vi "XYgraphBuffer.vi"(8 "Size":i32=100, 11 "X-Y Coord":dbl[](array[numeric])=[0.0, 0.0]) -> (3 "ToXYGraph":T1(array[cluster]))   [LabVIEW 2010, in "kevLib2011.lvlib"]
uses:
  kevLib2011.lvlib
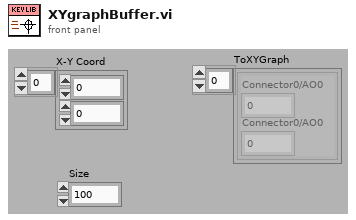
[diagram p1: front panel]
types:
  T1 = cluster{"Connector0/AO0":dbl, "Connector0/AO0":dbl}[]
  T2 = cluster{"Connector0/AO0":dbl, "Connector0/AO0":dbl}
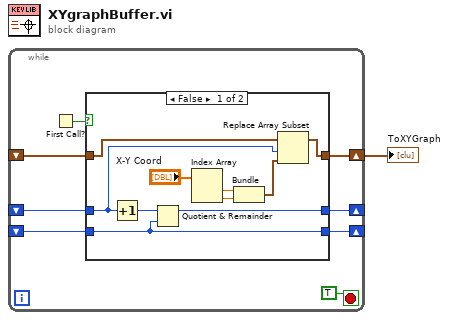
[diagram p0: block diagram]
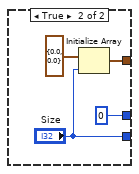
[diagram p2: hidden frame]
diagram:
  n1 = while {
    shift-right: [w8] -> w1
    shift-left: _ -> [w2]
    shift-right: [w6] -> _
    shift-left: _ -> [w4]
    shift-right: [w5] -> _
    shift-left: _ -> [w3]
    stop <- TRUE stop-if-true
    n2 = First Call?() -> (First Call?: T/F=w9:bool)
    n3 = case shown="False" w9 {
      tunnel: [w10 w22] -> w8
      tunnel: [w18 0] -> w6
      tunnel: [w17 "Size"] -> w5
      tunnel: w4 -> [w15 _]
      tunnel: w3 -> [w17 _]
      tunnel: w2 -> [w16 _]
      frame False {
        n4 = Increment(x=w15) -> (x+1=w19:i32)
        n5 = Quotient & Remainder(x=w19, y=w17) -> (x-y*floor(x/y)=w18:i32)  [unwired: 1 out]
        n6 = Index Array(array="X-Y Coord") -> (element #1=w12:dbl, element #2=w13:dbl)  [unwired: 2 in]
        n7 = Bundle("Waveform"=w12, "Waveform"=w13) -> (w11:cluster{"Waveform":dbl, "Waveform":dbl})  [unwired: 1 in]
        n8 = Replace Array Subset(array=w16, new element=w11, index=w15) -> (w10:T1)
      }
      frame True {
        n9 = Initialize Array(T2 {"Connector0/AO0"=0.0, "Connector0/AO0"=0.0} ("output cluster"), "Size") -> (w22:T1)
      }
    }
  }
  "ToXYGraph" <- w1
